vi "create queues.vi"(8 "error in (no error)":errorcluster, 11 "create if not found? (T)":bool=TRUE) -> (0 "error out":errorcluster, 1 "i2c queue out":refnum<queue>, 2 "power monitor queue out":refnum<queue>, 3 "image queue out":refnum<queue>, 5 "register monitor queue out":refnum<queue>)   [LabVIEW 2025, in "Automotive Vision.lvclass"]
uses:
  Automotive Vision.lvclass
  regitster_value.ctl
  power.ctl
  image.ctl
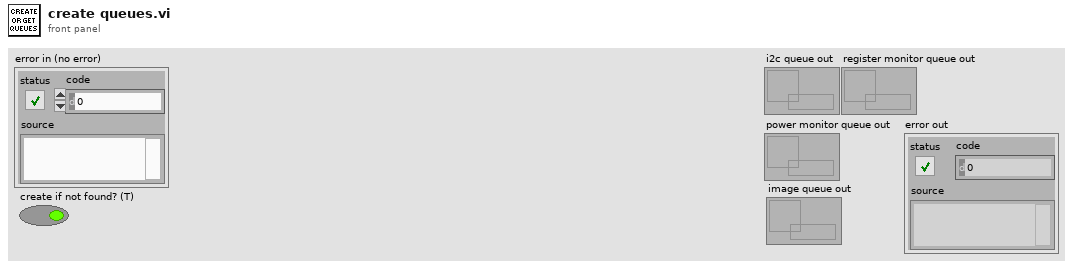
[diagram p1: front panel]
types:
  T1 = typedef "Automotive Vision.lvclass/image.ctl" = cluster{"Frame ID":u32, "Data":u8[]}
  T2 = typedef "Automotive Vision.lvclass/power.ctl" = cluster{"Voltage":dbl, "Current":dbl}
  T3 = typedef "Automotive Vision.lvclass/regitster_value.ctl" = cluster{"Source":u8, "Address":u16, "Value":u16}
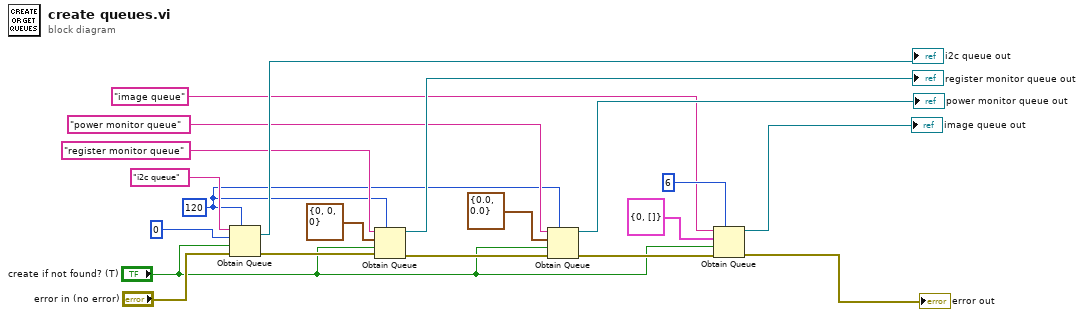
[diagram p0: block diagram]
diagram:
  w8 = 120 ("max queue size (-1, unlimited)")
  n1 = Obtain Queue(max queue size (-1, unlimited)=w8, name (unnamed)="i2c queue", element data type=u64 0, create if not found? (T)="create if not found? (T)", error in (no error)="error in (no error)") -> (queue out=→"i2c queue out":refnum<queue>, error out=w16:errorcluster)  [unwired: 1 out]
  n2 = Obtain Queue(max queue size (-1, unlimited)=w8, name (unnamed)="register monitor queue", element data type=T3 {"Source"=0, "Address"=0, "Value"=0} ("Register Value"), create if not found? (T)="create if not found? (T)", error in (no error)=w16) -> (queue out=→"register monitor queue out":refnum<queue>, error out=w12:errorcluster)  [unwired: 1 out]
  n3 = Obtain Queue(max queue size (-1, unlimited)=w8, name (unnamed)="power monitor queue", element data type=T2 {"Voltage"=0.0, "Current"=0.0} ("Power"), create if not found? (T)="create if not found? (T)", error in (no error)=w12) -> (queue out=→"power monitor queue out":refnum<queue>, error out=w7:errorcluster)  [unwired: 1 out]
  n4 = Obtain Queue(max queue size (-1, unlimited)=6, name (unnamed)="image queue", element data type=T1 {"Frame ID"=0, "Data"=[]} ("Image"), create if not found? (T)="create if not found? (T)", error in (no error)=w7) -> (queue out=→"image queue out":refnum<queue>, error out=→"error out":errorcluster)  [unwired: 1 out]
